vi "Special Read N Byte.vi"(8 "error in (no error)":errorcluster, 9 "Timeout (10000ms)":u32=10000, 10 "Read Count (1024)":u32=1024, 11 "VISA resource name":refnum<visa-resource-name>) -> (0 "error out":errorcluster, 1 "Return Count":u32, 2 "Read Buffer":string, 3 "VISA resource name out":refnum<visa-resource-name>)   [LabVIEW 2009, in "DSO1K.lvlib"]
doc: "Read N bytes that you set for this vi."
uses:
  <instrlib>/DSO1K/DSO1K.lvlib
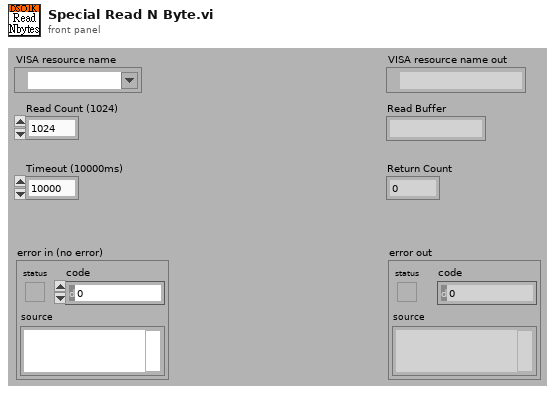
[diagram p1: front panel]
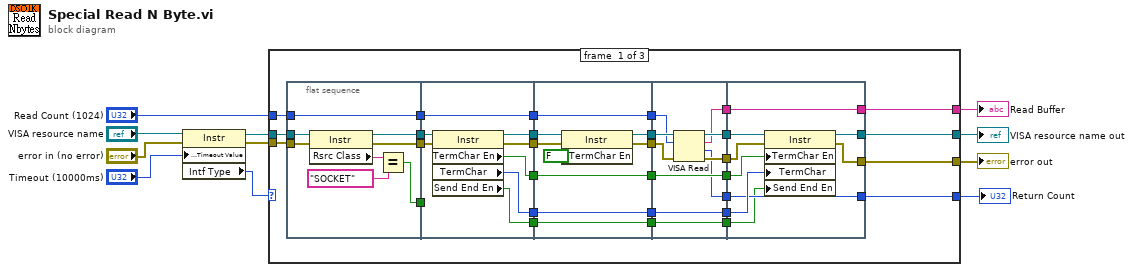
[diagram p0: block diagram]
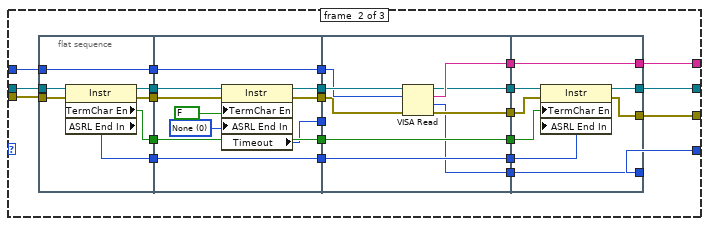
[diagram p2: hidden frame]
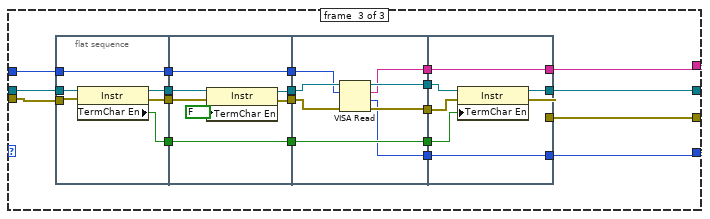
[diagram p3: hidden frame]
diagram:
  n1 = property class="Instr"(reference="VISA resource name", error in="error in (no error)", "General Settings:Timeout Value"="Timeout (10000ms)") -> (reference out=w7:refnum<visa-resource-name>, error out=w4:errorcluster, "Intf Type"=w1:u16)
  n2 = case shown="4, Default" w1 {
    tunnel: "Read Count (1024)" -> [w26 w97 w162]
    tunnel: [w28 w96 w159] -> w10
    tunnel: [w27 w95 w158] -> w9
    tunnel: [w29 w94 w147] -> w8
    tunnel: w7 -> [w25 w93 w161]
    tunnel: w4 -> [w24 w92 w160]
    tunnel: [w16 w87 w145] -> w2
    frame #0 {
      n3 = flat-sequence {
        tunnel: w26 -> [w49]
        tunnel: w24 -> [w47]
        tunnel: w25 -> [w48]
        tunnel: [w43] -> w23
        tunnel: [w44] -> w22
        tunnel: [w49] -> w21
        tunnel: [w42] -> w20
        tunnel: [w55] -> w41
        tunnel: [w54] -> w40
        tunnel: [w53] -> w39
        tunnel: [w52] -> w38
        tunnel: w23 -> [w57]
        tunnel: w22 -> [w56]
        tunnel: w21 -> [w53]
        tunnel: w20 -> [_]
        tunnel: [w51] -> w19
        tunnel: [w50] -> w12
        tunnel: w41 -> [w66]
        tunnel: w40 -> [w65]
        tunnel: [w64] -> w37
        tunnel: [w63] -> w36
        tunnel: [w62] -> w35
        tunnel: w39 -> [w62]
        tunnel: [w61] -> w34
        tunnel: w38 -> [w61]
        tunnel: w19 -> [w60]
        tunnel: [w60] -> w17
        tunnel: [w58] -> w13
        tunnel: w12 -> [w58]
        tunnel: w37 -> [w76]
        tunnel: w36 -> [w70]
        tunnel: w35 -> [w75]
        tunnel: [w74] -> w33
        tunnel: [w73] -> w32
        tunnel: [w72] -> w31
        tunnel: w34 -> [w72]
        tunnel: [w71] -> w30
        tunnel: [w69] -> w18
        tunnel: w17 -> [w69]
        tunnel: [w68] -> w15
        tunnel: [w67] -> w14
        tunnel: w13 -> [w67]
        tunnel: w33 -> [w85]
        tunnel: w32 -> [w80]
        tunnel: [w84] -> w28
        tunnel: [w81] -> w27
        tunnel: w31 -> [w83]
        tunnel: [w82] -> w29
        tunnel: w30 -> [w82]
        tunnel: w18 -> [w79]
        tunnel: [w78] -> w16
        tunnel: w15 -> [w78]
        tunnel: w14 -> [w77]
        frame #0 {
          n4 = property class="Instr"(reference=w48, error in=w47) -> (reference out=w43:refnum<visa-resource-name>, error out=w44:errorcluster, "Rsrc Class"=w46:string)
          n5 = Equal?(x=w46, y="SOCKET") -> (x = y?=w42:bool)
        }
        frame #1 {
          n6 = property class="Instr"(reference=w57, error in=w56) -> (reference out=w55:refnum<visa-resource-name>, error out=w54:errorcluster, "TermChar En"=w52:bool, "TermChar"=w51:u8, "Send End En"=w50:bool)
        }
        frame #2 {
          n7 = property class="Instr"(reference=w66, error in=w65, "TermChar En"=FALSE ("Message Based Settings:Termination Character Enable")) -> (reference out=w64:refnum<visa-resource-name>, error out=w63:errorcluster)
        }
        frame #3 {
          n8 = VISA Read(VISA resource name=w76, byte count=w75, error in (no error)=w70) -> (VISA resource name out=w74:refnum<visa-resource-name>, read buffer=w71:string, return count=w68:u32, error out=w73:errorcluster)
        }
        frame #4 {
          n9 = property class="Instr"(reference=w85, error in=w80, "TermChar En"=w83, "TermChar"=w79, "Send End En"=w77) -> (reference out=w84:refnum<visa-resource-name>, error out=w81:errorcluster)
        }
      }
    }
    frame #1 {
      n10 = flat-sequence {
        tunnel: w93 -> [w116]
        tunnel: w92 -> [w115]
        tunnel: [w114] -> w109
        tunnel: [w113] -> w108
        tunnel: [w112] -> w107
        tunnel: w97 -> [w112]
        tunnel: [w111] -> w106
        tunnel: [w110] -> w91
        tunnel: w109 -> [w125]
        tunnel: w108 -> [w124]
        tunnel: [w123] -> w105
        tunnel: [w122] -> w104
        tunnel: [w121] -> w103
        tunnel: w107 -> [w121]
        tunnel: [w120] -> w102
        tunnel: w106 -> [w120]
        tunnel: w91 -> [w119]
        tunnel: [w119] -> w90
        tunnel: [w117] -> w86
        tunnel: w105 -> [w133]
        tunnel: w104 -> [w131]
        tunnel: w103 -> [w132]
        tunnel: [w127] -> w101
        tunnel: [w130] -> w100
        tunnel: [w135] -> w99
        tunnel: w102 -> [w135]
        tunnel: [w128] -> w98
        tunnel: w90 -> [w134]
        tunnel: [w134] -> w89
        tunnel: [w129] -> w88
        tunnel: w86 -> [_]
        tunnel: w101 -> [w143]
        tunnel: w100 -> [w138]
        tunnel: [w142] -> w96
        tunnel: [w139] -> w95
        tunnel: w99 -> [w141]
        tunnel: [w140] -> w94
        tunnel: w98 -> [w140]
        tunnel: w89 -> [w137]
        tunnel: w88 -> [w136]
        tunnel: [w136] -> w87
        frame #0 {
          n11 = property class="Instr"(reference=w116, error in=w115) -> (reference out=w114:refnum<visa-resource-name>, error out=w113:errorcluster, "TermChar En"=w111:bool, "ASRL End In"=w110:u16)
        }
        frame #1 {
          w118 = u16 0 items=["None", "Last Bit", "TermChar"] ("Serial Settings:End Mode for Reads")
          n12 = property class="Instr"(reference=w125, error in=w124, "TermChar En"=FALSE ("Message Based Settings:Termination Character Enable"), "ASRL End In"=w118) -> (reference out=w123:refnum<visa-resource-name>, error out=w122:errorcluster, "Timeout"=w117:u32)
        }
        frame #2 {
          n13 = VISA Read(VISA resource name=w133, byte count=w132, error in (no error)=w131) -> (VISA resource name out=w127:refnum<visa-resource-name>, read buffer=w128:string, return count=w129:u32, error out=w130:errorcluster)
        }
        frame #3 {
          n14 = property class="Instr"(reference=w143, error in=w138, "TermChar En"=w141, "ASRL End In"=w137) -> (reference out=w142:refnum<visa-resource-name>, error out=w139:errorcluster)
        }
      }
    }
    frame #2 {
      n15 = flat-sequence {
        tunnel: [w169] -> w157
        tunnel: [w168] -> w155
        tunnel: [w167] -> w153
        tunnel: [w166] -> w151
        tunnel: w162 -> [w167]
        tunnel: w161 -> [w165]
        tunnel: w160 -> [w164]
        tunnel: w157 -> [w173]
        tunnel: [w172] -> w156
        tunnel: w155 -> [w170]
        tunnel: [w171] -> w154
        tunnel: w153 -> [w176]
        tunnel: [w176] -> w152
        tunnel: w151 -> [w175]
        tunnel: [w175] -> w150
        tunnel: w156 -> [w180]
        tunnel: w154 -> [w183]
        tunnel: w152 -> [w179]
        tunnel: [w184] -> w163
        tunnel: w150 -> [w184]
        tunnel: [w181] -> w149
        tunnel: [w182] -> w148
        tunnel: [w178] -> w146
        tunnel: [w177] -> w144
        tunnel: [w191] -> w159
        tunnel: [w189] -> w158
        tunnel: w163 -> [w190]
        tunnel: w149 -> [w188]
        tunnel: w148 -> [w187]
        tunnel: [w186] -> w147
        tunnel: w146 -> [w186]
        tunnel: [w185] -> w145
        tunnel: w144 -> [w185]
        frame #0 {
          n16 = property class="Instr"(reference=w165, error in=w164) -> (reference out=w169:refnum<visa-resource-name>, error out=w168:errorcluster, "TermChar En"=w166:bool)
        }
        frame #1 {
          n17 = property class="Instr"(reference=w173, error in=w170, "TermChar En"=FALSE ("Message Based Settings:Termination Character Enable")) -> (reference out=w172:refnum<visa-resource-name>, error out=w171:errorcluster)
        }
        frame #2 {
          n18 = VISA Read(VISA resource name=w180, byte count=w179, error in (no error)=w183) -> (VISA resource name out=w181:refnum<visa-resource-name>, read buffer=w178:string, return count=w177:u32, error out=w182:errorcluster)
        }
        frame #3 {
          n19 = property class="Instr"(reference=w188, error in=w187, "TermChar En"=w190) -> (reference out=w191:refnum<visa-resource-name>, error out=w189:errorcluster)
        }
      }
    }
  }
  "Read Buffer" <- w8
  "VISA resource name out" <- w10
  "error out" <- w9
  "Return Count" <- w2
